vi "Find Object Item Locations by Names.vi"(5 "Insertion point if not found":bool, 6 "Only return first found":bool, 7 "Item Names <JSON>":string[](array[string]), 8 "error in (no error)":errorcluster, 10 "Object Offset":i32, 11 "JSON":string) -> (0 "error out":errorcluster, 1 "Items":T1[](array[typedef]))   [LabVIEW 2019, in "JSONtext.lvlib"]
uses:
  JSONtext.lvlib
  Parsing/Found Items.ctl
  Parsing/Parsing State.ctl
  Parsing/Advance past Line Ending.vi
  Parsing/Advance past String.vi
  Parsing/Advance past Number.vi
  Parsing/Advance past Array.vi
  Parsing/Advance past Object.vi
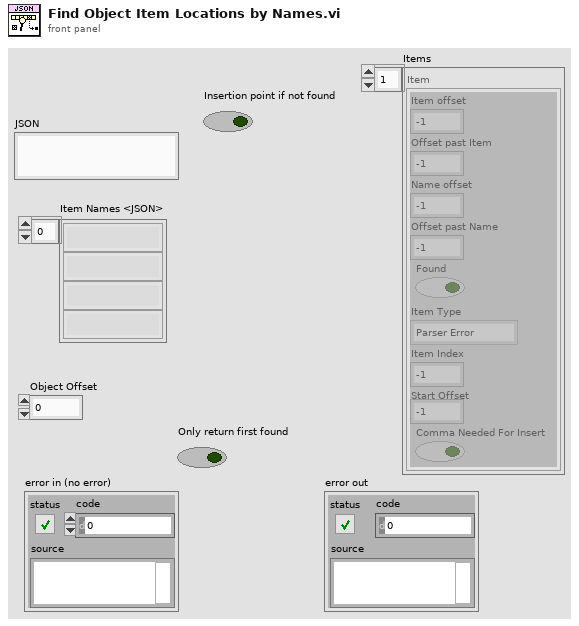
[diagram p1: front panel]
types:
  T1 = typedef "JSONtext.lvlib/Found Items.ctl" = cluster{"Item offset":i32, "Offset past Item":i32, "Name offset":i32, "Offset past Name":i32, "Found":bool, "Item Type":T2, "Item Index":i32, "Start Offset":i32, "Comma Needed For Insert":bool}
  T2 = typedef "JSONtext.lvlib/Parsing State.ctl" = enum16{"Parser Error", "Object", "Array", "String", "Number/Other", "Leading Whitespace", "Object end", "Array end", "Value end"}
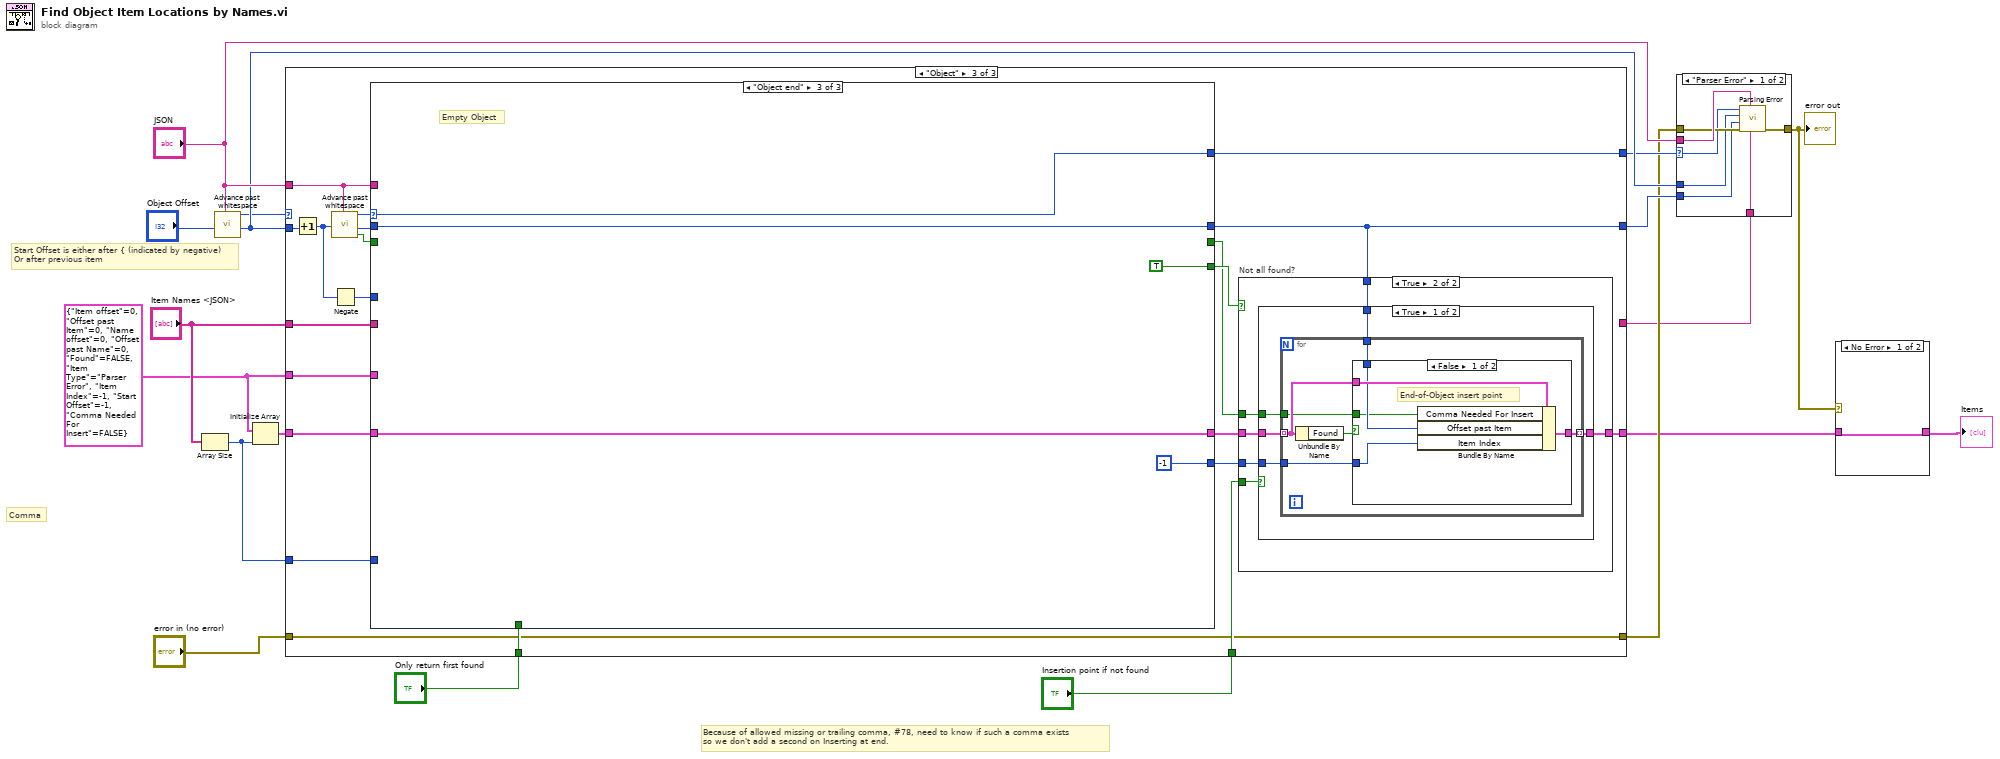
[diagram p0: block diagram]
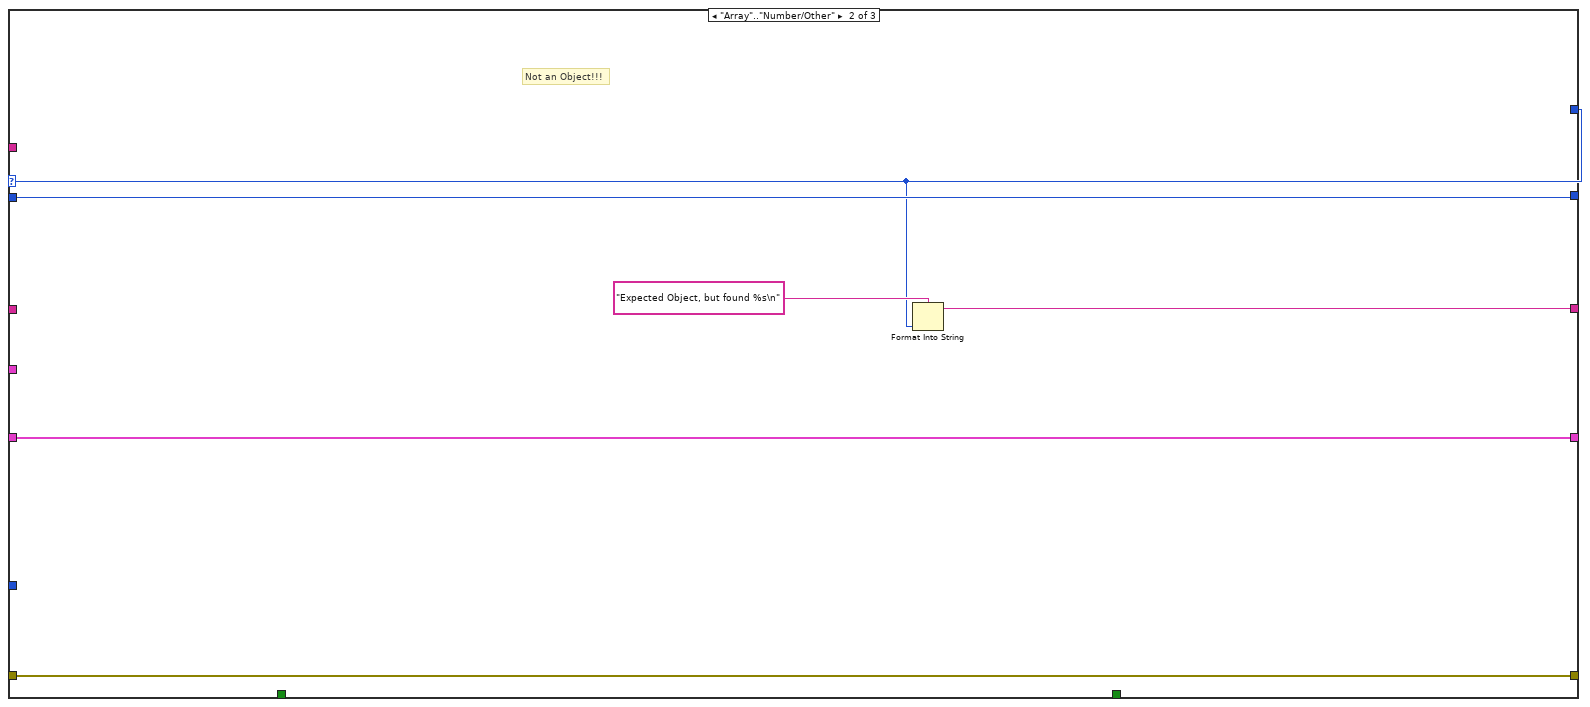
[diagram p3: hidden frame]
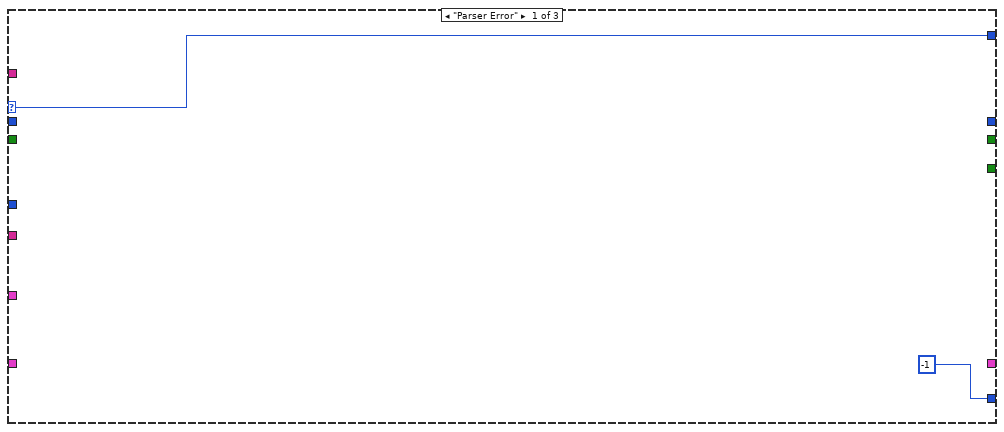
[diagram p4: hidden frame]
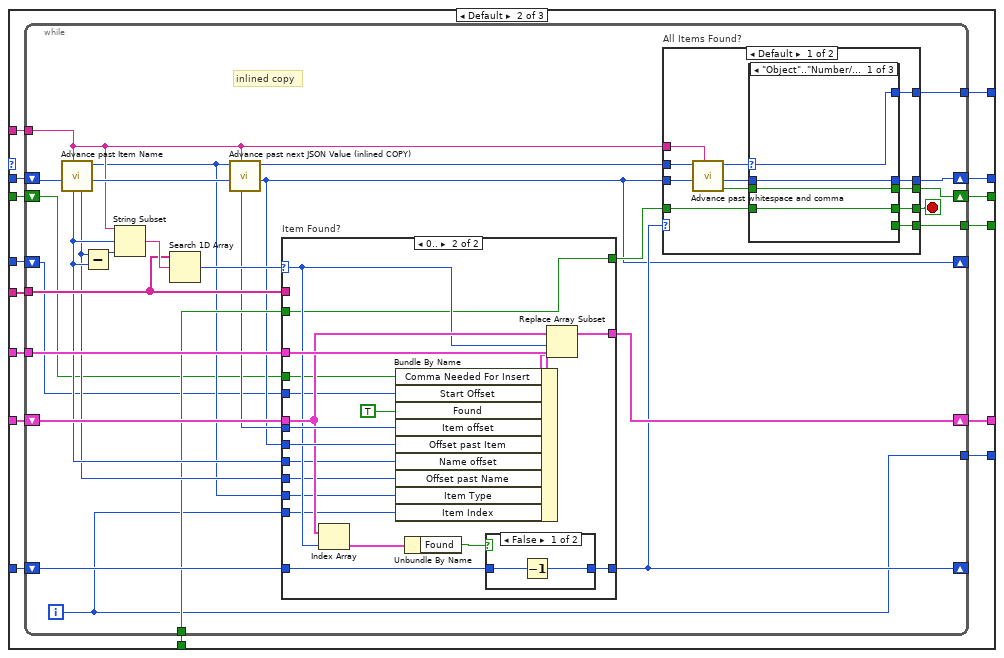
[diagram p5: hidden frame]
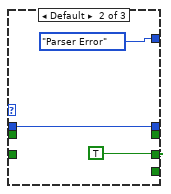
[diagram p8: hidden frame]
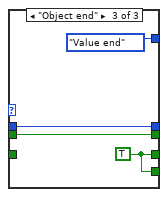
[diagram p9: hidden frame]
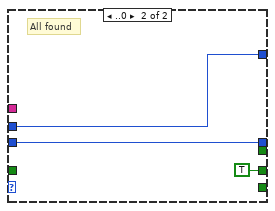
[diagram p10: hidden frame]
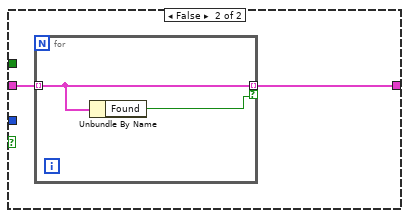
[diagram p13: hidden frame]
diagram:
  w15 = T1 {"Item offset"=0, "Offset past Item"=0, "Name offset"=0, "Offset past Name"=0, "Found"=FALSE, "Item Type"=enum."Parser Error", "Item Index"=-1, "Start Offset"=-1, "Comma Needed For Insert"=FALSE}
  # "Because of allowed missing or trailing comma, #78, need to know if such a comma exists \nso we don't add a second on Inserting at end."
  # "Comma"
  # "Start Offset is either after { (indicated by negative)\nOr after previous item"
  n1 = Array Size(array="Item Names <JSON>") -> (size(s)=w14:i32)
  n2 = call "Advance past whitespace.vi"("JSON"="JSON", "Offset"="Object Offset") -> ("Offset of first non-whitespace"=w11:i32, "Parser State"=w10:T2)  [unwired: 7 in, 1 out]
  n3 = Initialize Array(w15, w14) -> (w16:T1[])
  n4 = case shown="\"Object\"" w10 {
    selector: w10 -> [w19 w24 _]
    tunnel: "Item Names <JSON>" -> [_ _ w49]
    tunnel: w16 -> [w22 w28 w48]
    tunnel: w15 -> [_ _ w47]
    tunnel: w14 -> [_ _ w46]
    tunnel: [w22 w28 w43] -> w2
    tunnel: "JSON" -> [_ _ w37]
    tunnel: [w20 w26 w42] -> w12
    tunnel: w11 -> [w20 w26 w33]
    tunnel: [w19 w24 w41] -> w9
    tunnel: "Only return first found" -> [_ _ w40]
    tunnel: "Insertion point if not found" -> [_ _ w39]
    tunnel: "error in (no error)" -> [w21 w27 w38]
    tunnel: [w21 w27 w38] -> w5
    tunnel: [_ w23 _] -> w1
    frame "Parser Error", Default {
      # "Not an Object!!!"
    }
    frame "Array".."Number/Other" {
      # "Not an Object!!!"
      n5 = Format Into String(format string="Expected Object, but found %s\n", w24) -> (resulting string=w23:string)  [unwired: 2 in, 1 out]
    }
    frame "Object" {
      n6 = Increment(x=w33) -> (x+1=w32:i32)
      n7 = call "Advance past whitespace.vi"("JSON"=w37, "Offset"=w32) -> ("Comma Not Found"=w29:bool, "Offset of first non-whitespace"=w36:i32, "Parser State"=w35:T2)  [unwired: 7 in]
      n8 = Negate(x=w32) -> (-x=w31:i32)
      n9 = case shown="\"Object end\"" w35 {
        selector: w35 -> [w51 _ w148]
        tunnel: w36 -> [_ w66 w147]
        tunnel: w49 -> [_ w65 _]
        tunnel: w48 -> [_ w64 w146]
        tunnel: w47 -> [_ w63 _]
        tunnel: w46 -> [_ w62 _]
        tunnel: [_ w61 w146] -> w45
        tunnel: [_ w60 TRUE] -> w44
        tunnel: w37 -> [_ w59 _]
        tunnel: [_ w58 w147] -> w42
        tunnel: [w51 w57 w148] -> w41
        tunnel: w40 -> [_ w56 _]
        tunnel: [-1 w55 -1] -> w34
        tunnel: w31 -> [_ w54 _]
        tunnel: [_ w53 _] -> w30
        tunnel: w29 -> [_ w52 _]
        frame "Parser Error" {
        }
        frame Default {
          n10 = while {
            shift-right: [w94] -> w58
            shift-left: w66 -> [w91]
            tunnel: w59 -> [w88]
            tunnel: [w92] -> w57
            tunnel: w65 -> [w83]
            tunnel: w63 -> [w85]
            shift-right: [w81] -> w61
            shift-left: w64 -> [w82]
            shift-right: [w79] -> _
            shift-left: w62 -> [w80]
            tunnel: [w78] -> w60
            tunnel: w56 -> [w75]
            tunnel: [w71] -> w55
            shift-right: [w70] -> _
            shift-left: w54 -> [w69]
            shift-right: [w68] -> w53
            shift-left: w52 -> [w67]
            i -> [w71]
            stop <- w93 stop-if-true
            # "inlined copy"
            n11 = call "Advance past Item Name.vi"("JSON"=w88, "Offset"=w91) -> ("Offset past colon"=w89:i32, "State"=w72:T2, "Offset past Name"=w76:i32, "Name start out"=w77:i32)  [unwired: 6 in]
            n12 = Subtract(x=w76, y=w77) -> (x-y=w87:i32)
            n13 = String Subset(string=w88, offset (0)=w77, length (rest)=w87) -> (substring=w86:string)
            n14 = Search 1D Array(1D array=w83, element=w86) -> (index of element=w84:i32)  [unwired: 1 in]
            n15 = call "Advance past next JSON Value (inlined COPY).vi"("JSON"=w88, "Offset"=w89, "State"=w72) -> ("Offset"=w70:i32, "State"=w90:T2, "Value start"=w73:i32)  [unwired: 4 in, 2 out]
            n16 = case "Item Found?" shown="0.." w84 {
              selector: w84 -> [_ w109]
              tunnel: w85 -> [_ w115]
              tunnel: w73 -> [_ w113]
              tunnel: w70 -> [_ w112]
              tunnel: w83 -> [_ _]
              tunnel: w82 -> [w96 w110]
              tunnel: [w96 w108] -> w81
              tunnel: w80 -> [w95 w105]
              tunnel: [w95 w104] -> w79
              tunnel: w77 -> [_ w103]
              tunnel: w76 -> [_ w102]
              tunnel: w75 -> [_ w101]
              tunnel: [_ w101] -> w74
              tunnel: w72 -> [_ w100]
              tunnel: w71 -> [_ w99]
              tunnel: w69 -> [_ w98]
              tunnel: w67 -> [_ w97]
              frame Default {
              }
              frame 0.. {
                n17 = Index Array(array=w110, index=w109) -> (element=w107:T1)
                n18 = Bundle By Name(cluster=w115, "Comma Needed For Insert"=w97, "Start Offset"=w98, "Found"=TRUE, "Item offset"=w113, "Offset past Item"=w112, "Name offset"=w103, "Offset past Name"=w102, "Item Type"=w100, "Item Index"=w99) -> (w111:T1)
                n19 = Unbundle By Name(w107) -> ("Found"=w106:bool)
                n20 = case shown="False" w106 {
                  tunnel: w105 -> [w117 w118]
                  tunnel: [w116 w118] -> w104
                  frame False {
                    n21 = Decrement(x=w117) -> (x-1=w116:i32)
                  }
                  frame True {
                  }
                }
                n22 = Replace Array Subset(array=w110, new element=w111, index=w109) -> (w108:T1[])
              }
            }
            n23 = case "All Items Found?" shown="Default" w79 {
              tunnel: [w129 w143] -> w94
              tunnel: [w128 TRUE] -> w93
              tunnel: [w127 w144] -> w92
              tunnel: w90 -> [w122 w144]
              tunnel: w70 -> [w125 w143]
              tunnel: w88 -> [w126 _]
              tunnel: [w123 _] -> w78
              tunnel: w74 -> [w121 _]
              tunnel: [w119 _] -> w68
              frame Default {
                n24 = call "Advance past whitespace and comma.vi"("JSON"=w126, "Offset"=w125, "State in"=w122) -> ("Comma Not Found"=w120:bool, "Offset past match"=w124:i32, "State"=w130:T2)  [unwired: 6 in]
                n25 = case shown="\"Object\"..\"Number/Other\"" w130 {
                  selector: w130 -> [w132 _ _]
                  tunnel: [w133 TRUE w140] -> w128
                  tunnel: [w132 Parsing_State."Parser Error" Parsing_State."Value end"] -> w127
                  tunnel: w124 -> [w134 w135 w139]
                  tunnel: [w134 w135 w139] -> w129
                  tunnel: [_ _ w140] -> w123
                  tunnel: w121 -> [w133 _ _]
                  tunnel: w120 -> [w131 _ w138]
                  tunnel: [w131 _ w138] -> w119
                  frame "Object".."Number/Other" {
                  }
                  frame Default {
                  }
                  frame "Object end" {
                    w140 = TRUE
                  }
                }
              }
              frame ..0 {
                # "All found"
              }
            }
          }
        }
        frame "Object end" {
          # "Empty Object"
        }
      }
      n26 = case "Not all found?" shown="True" w44 {
        tunnel: w45 -> [w150 w156]
        tunnel: [w150 w155] -> w43
        tunnel: w42 -> [_ w154]
        tunnel: w39 -> [_ w153]
        tunnel: w34 -> [_ w152]
        tunnel: w30 -> [_ w151]
        frame False {
        }
        frame True {
          n27 = case shown="True" w153 {
            tunnel: w156 -> [w162 w176]
            tunnel: [w161 w175] -> w155
            tunnel: w154 -> [w160 _]
            tunnel: w152 -> [w159 _]
            tunnel: w151 -> [w157 _]
            frame True {
              n28 = Increment(x=w159) -> (x+1=w158:i32)
              n29 = for {
                tunnel: w162 -> [w166] mode=indexing
                tunnel: [w167] -> w161 mode=indexing
                tunnel: w160 -> [w165]
                tunnel: w158 -> [w164]
                tunnel: w157 -> [w163]
                n30 = Unbundle By Name(w166) -> ("Found"=w168:bool)
                n31 = case shown="False" w168 {
                  tunnel: [w172 w174] -> w167
                  tunnel: w166 -> [w173 w174]
                  tunnel: w165 -> [w171 _]
                  tunnel: w164 -> [w170 _]
                  tunnel: w163 -> [w169 _]
                  frame False {
                    # "End-of-Object insert point"
                    n32 = Bundle By Name(cluster=w173, "Comma Needed For Insert"=w169, "Offset past Item"=w171, "Item Index"=w170) -> (w172:T1)
                  }
                  frame True {
                  }
                }
              }
            }
            frame False {
              n33 = for {
                tunnel: w176 -> [w178] mode=indexing
                tunnel: [w178] -> w175 mode=indexing if=w177
                n34 = Unbundle By Name(w178) -> ("Found"=w177:bool)
              }
            }
          }
        }
      }
    }
  }
  n35 = case shown="\"Parser Error\"" w9 {
    selector: w9 -> [w180 _]
    tunnel: "JSON" -> [w185 _]
    tunnel: w5 -> [w184 w186]
    tunnel: [w183 w186] -> w4
    tunnel: w11 -> [w182 _]
    tunnel: w12 -> [w181 _]
    tunnel: w1 -> [w179 _]
    frame "Parser Error" {
      n36 = call "Parsing Error.vi"("initial string"=w179, "JSON"=w185, "error in (no error)"=w184, "Offset past match"=w181, "Value start"=w182, "State"=w180) -> ("error out"=w183:errorcluster)  [unwired: 5 in]
    }
    frame Default {
    }
  }
  "error out" <- w4
  n37 = case shown="No Error" w4 {
    tunnel: [w187 _] -> w3
    tunnel: w2 -> [w187 _]
    frame No Error {
    }
    frame Error {
    }
  }
  "Items" <- w3
